vi "validate line configuration.vi"(7 "warn?":bool, 11 "line in":T1) -> (1 "valid?":bool, 3 "line out":T1, 5 "still warn?":bool)   [LabVIEW 2013, in "Scan Engine editor node.lvclass"]
uses:
  Scan Engine editor node.lvclass
  table line.ctl
  <vilib>/NI/Tag Bus Module Framework/channel/TBM channel.lvclass
  <vilib>/NI/Tag Bus/tag/tag descriptor.lvclass/tag descriptor.ctl
  <vilib>/NI/Tag Bus/tag/read tag name.vi
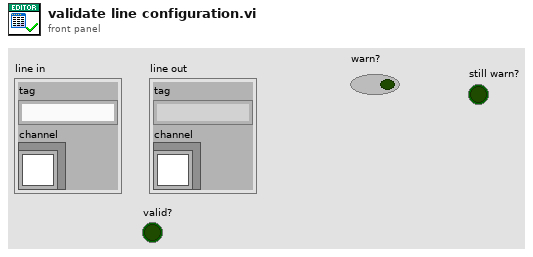
[diagram p1: front panel]
types:
  T1 = typedef "Scan Engine editor node.lvclass/table line.ctl" = cluster{"tag":string, "channel":refnum<class "TBM channel.lvclass">}
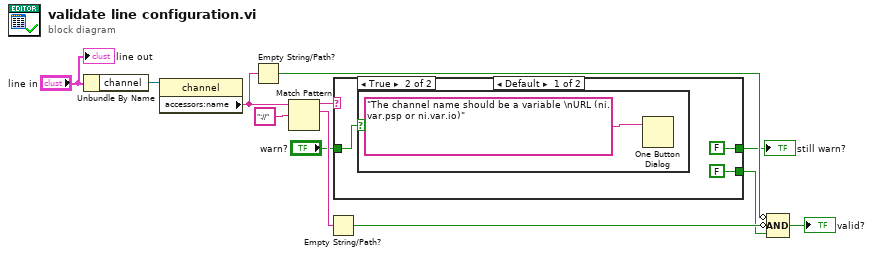
[diagram p0: block diagram]
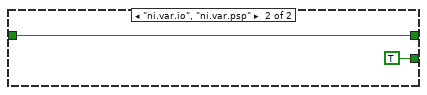
[diagram p3: hidden frame]
diagram:
  n1 = Unbundle By Name("line in") -> ("channel"=w11:refnum<class "TBM channel.lvclass">)
  n2 = property class="channel"(reference=w11) -> ("accessors:name"=w9:string)  [unwired: 1 in, 2 out]
  n3 = Empty String/Path?(string/path=w9) -> (empty?=w10:bool)
  n4 = Match Pattern(string=w9, regular expression="://") -> (before substring=w4:string, match substring=w7:string)  [unwired: 1 in, 2 out]
  n5 = Empty String/Path?(string/path=w7) -> (empty?=w5:bool)
  n6 = case shown="Default" w4 {
    tunnel: [FALSE TRUE] -> w3
    tunnel: [FALSE ("warn?") w17] -> w2
    tunnel: "warn?" -> [w13 w17]
    frame Default {
      n7 = case shown="True" w13 {
        frame False {
        }
        frame True {
          n8 = One Button Dialog(message="The channel name should be a variable \nURL (ni.var.psp or ni.var.io)") -> ()  [unwired: 1 in, 1 out]
        }
      }
    }
    frame "ni.var.io", "ni.var.psp" {
    }
  }
  "still warn?" <- w2
  n9 = Compound Arithmetic op=AND(invert w10, invert w5, w3) -> (→"valid?":bool)
  "line out" <- "line in"
